vi "Get Frame Signals.vi"(6 "CAN:Frame Type":T1=enum."All", 8 "error in":errorcluster, 9 "Parent Tag":string, 10 "Tree Reference":refnum<vi>, 11 "Frms":refnum<k21>[](array[refnum])) -> (0 "error out":errorcluster, 2 "Tree Reference Out":refnum<vi>)   [LabVIEW 2023, in "J1939 Addon System Explorer.lvlib"]
uses:
  J1939 Addon System Explorer.lvlib
  Types/CAN Frame Filter.ctl
  <resource>/objmgr/xnet.rc
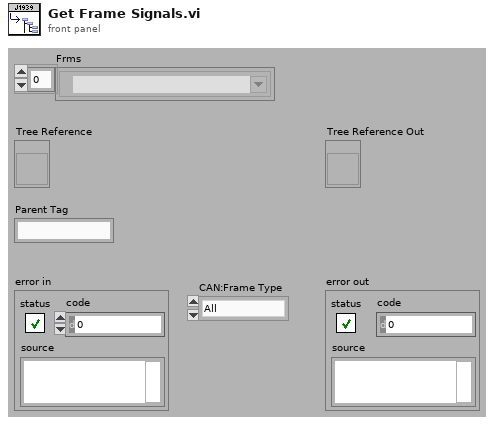
[diagram p1: front panel]
types:
  T1 = typedef "J1939 Addon System Explorer.lvlib/CAN Frame Filter.ctl" = enum16{"Cyclic Data", "Event Data", "Cyclic/Event", "All"}
  T2 = enum16{"open", "replace", "create", "open or create", "replace or create", "replace or create with confirmation"}
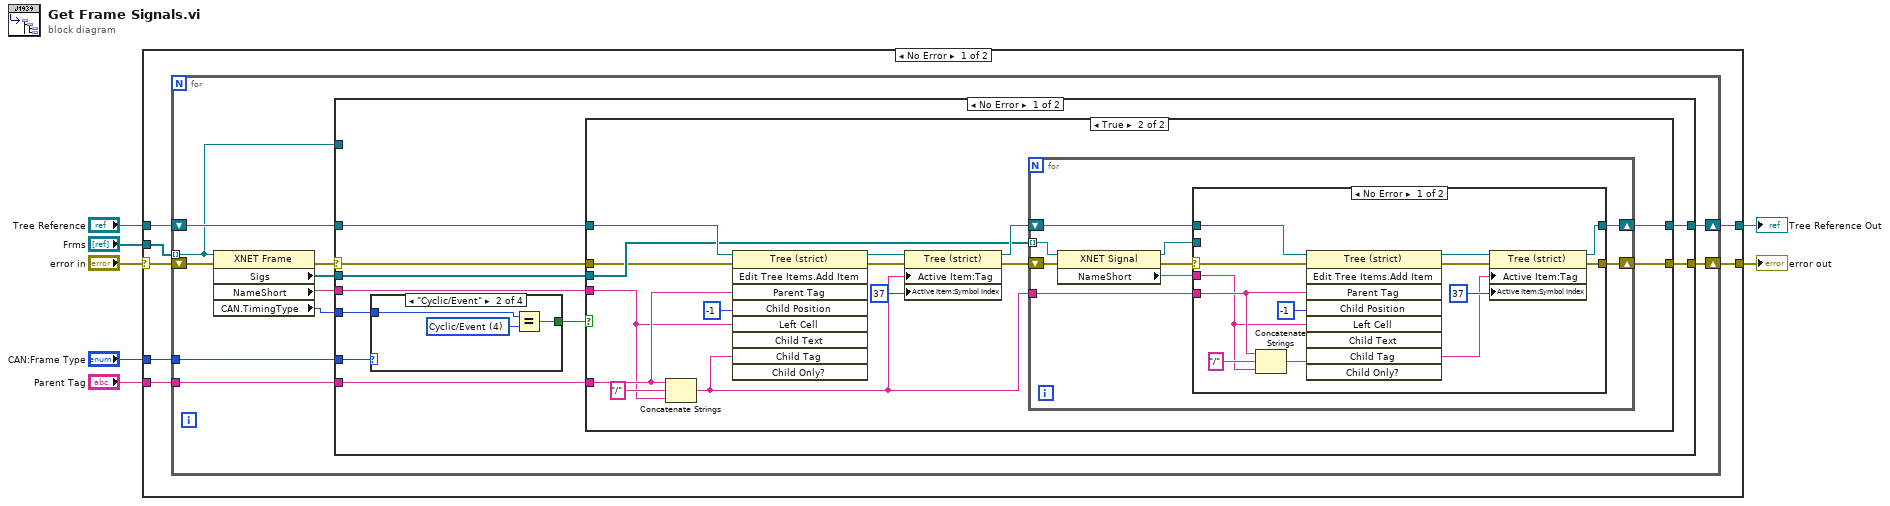
[diagram p0: block diagram]
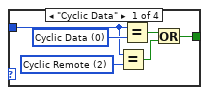
[diagram p2: hidden frame]
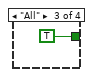
[diagram p3: hidden frame]
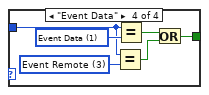
[diagram p4: hidden frame]
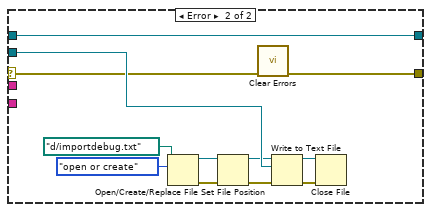
[diagram p6: hidden frame]
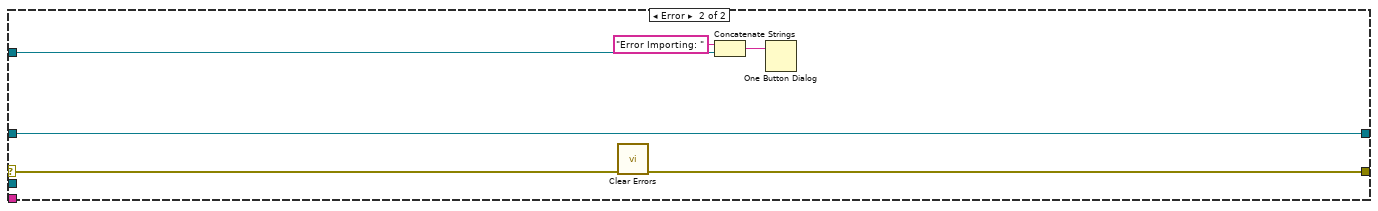
[diagram p7: hidden frame]
diagram:
  n1 = case shown="No Error" "error in" {
    selector: "error in" -> [w11 w109]
    tunnel: [w14 w109] -> w7
    tunnel: "Frms" -> [w9 _]
    tunnel: "Tree Reference" -> [w13 w108]
    tunnel: "Parent Tag" -> [w12 _]
    tunnel: [w10 w108] -> w2
    tunnel: "CAN:Frame Type" -> [w8 _]
    frame No Error {
      n2 = for {
        tunnel: w9 -> [w17] mode=indexing
        shift-right: [w20] -> w14
        shift-left: w11 -> [w25]
        tunnel: w12 -> [w23]
        shift-right: [w22] -> w10
        shift-left: w13 -> [w24]
        tunnel: w8 -> [w16]
        n3 = property class="XNET Frame"(reference=w17, error in=w25) -> (error out=w18:errorcluster, "Sigs"=w21:refnum<k21>[], "NameShort"=w19:string, "CAN.TimingType"=w15:u32)  [unwired: 1 out]
        n4 = case shown="No Error" w18 {
          selector: w18 -> [w29 w104]
          tunnel: w24 -> [w35 w102]
          tunnel: w23 -> [w34 _]
          tunnel: [w33 w102] -> w22
          tunnel: w21 -> [w32 _]
          tunnel: [w31 w103] -> w20
          tunnel: w19 -> [w30 _]
          tunnel: w17 -> [_ w107]
          tunnel: w16 -> [w26 _]
          tunnel: w15 -> [w28 _]
          frame No Error {
            n5 = case shown="\"Cyclic/Event\"" w26 {
              tunnel: w28 -> [w38 w43 _ w49]
              tunnel: [w36 w42 TRUE w47] -> w27
              frame "Cyclic Data" {
                w40 = u32 2 items=["Cyclic Data", "Event Data", "Cyclic Remote", "Event Remote", "Cyclic/Event"] ("CAN:Timing Type")
                w41 = u32 0 items=["Cyclic Data", "Event Data", "Cyclic Remote", "Event Remote", "Cyclic/Event"] ("CAN:Timing Type")
                n6 = Equal?(x=w38, y=w40) -> (x = y?=w39:bool)
                n7 = Equal?(x=w38, y=w41) -> (x = y?=w37:bool)
                n8 = Or(x=w37, y=w39) -> (x .or. y?=w36:bool)
              }
              frame "Cyclic/Event" {
                w44 = u32 4 items=["Cyclic Data", "Event Data", "Cyclic Remote", "Event Remote", "Cyclic/Event"] ("CAN:Timing Type")
                n9 = Equal?(x=w43, y=w44) -> (x = y?=w42:bool)
              }
              frame "All" {
              }
              frame "Event Data" {
                w48 = u32 3 items=["Cyclic Data", "Event Data", "Cyclic Remote", "Event Remote", "Cyclic/Event"] ("CAN:Timing Type")
                w50 = u32 1 items=["Cyclic Data", "Event Data", "Cyclic Remote", "Event Remote", "Cyclic/Event"] ("CAN:Timing Type")
                n10 = Equal?(x=w49, y=w48) -> (x = y?=w46:bool)
                n11 = Equal?(x=w49, y=w50) -> (x = y?=w51:bool)
                n12 = Or(x=w51, y=w46) -> (x .or. y?=w47:bool)
              }
            }
            n13 = case shown="True" w27 {
              tunnel: w35 -> [w53 w68]
              tunnel: w34 -> [_ w65]
              tunnel: [w53 w64] -> w33
              tunnel: w32 -> [_ w57]
              tunnel: [w52 w56] -> w31
              tunnel: w30 -> [_ w55]
              tunnel: w29 -> [w52 w54]
              frame False {
              }
              frame True {
                n14 = Concatenate Strings(w65, "/" ("string"), w55) -> (w58:string)
                n15 = invoke on="Invoke Node" class="Tree (strict)" method="Edit Tree Items.Add Item"(reference=w68, error in=w54, "Parent Tag"=w65, "Child Position"=-1, "Left Cell"=w55, "Child Tag"=w58) -> (reference out=w61:refnum<vi>, error out=w62:errorcluster)  [unwired: 3 in, 7 out]
                n16 = property class="Tree (strict)"(reference=w61, error in=w62, "Active Item:Tag"=w58, "Active Item:Symbol Index"=37) -> (reference out=w59:refnum<vi>, error out=w60:errorcluster)
                n17 = for {
                  tunnel: w57 -> [w70] mode=indexing
                  shift-right: [w72] -> w56
                  shift-left: w60 -> [w77]
                  tunnel: w58 -> [w75]
                  shift-right: [w73] -> w64
                  shift-left: w59 -> [w76]
                  n18 = property class="XNET Signal"(reference=w70, error in=w77) -> (reference out=w69:refnum<k21>, error out=w71:errorcluster, "NameShort"=w74:string)
                  n19 = case shown="No Error" w71 {
                    selector: w71 -> [w78 w99]
                    tunnel: w76 -> [w89 w101]
                    tunnel: w75 -> [w87 _]
                    tunnel: w74 -> [w86 _]
                    tunnel: [w81 w101] -> w73
                    tunnel: [w79 w98] -> w72
                    tunnel: w69 -> [_ w100]
                    frame No Error {
                      n20 = Concatenate Strings(w87, "/" ("string"), w86) -> (w80:string)
                      n21 = invoke on="Invoke Node" class="Tree (strict)" method="Edit Tree Items.Add Item"(reference=w89, error in=w78, "Parent Tag"=w87, "Child Position"=-1, "Left Cell"=w86, "Child Tag"=w80) -> (reference out=w82:refnum<vi>, error out=w83:errorcluster)  [unwired: 3 in, 7 out]
                      n22 = property class="Tree (strict)"(reference=w82, error in=w83, "Active Item:Tag"=w80, "Active Item:Symbol Index"=37) -> (reference out=w81:refnum<vi>, error out=w79:errorcluster)
                    }
                    frame Error {
                      n23 = Open/Create/Replace File(file path (use dialog)=path "d:/importdebug.txt", operation (0:open)=T2."open or create") -> (refnum out=w95:refnum<file>, error out=w96:errorcluster)  [unwired: 4 in, 1 out]
                      n24 = Set File Position(refnum=w95, error in=w96) -> (refnum out=w94:refnum<file>, error out=w93:errorcluster)  [unwired: 2 in]
                      n25 = call <vilib>:"Clear Errors.vi"("error in (no error)"=w99) -> ("error out"=w98:errorcluster)  [unwired: 5 in, 1 out]
                      n26 = Write to Text File(file (use dialog)=w94, text=w100, error in=w93) -> (refnum out=w91:refnum<file>, error out=w92:errorcluster)  [unwired: 1 in, 1 out]
                      n27 = Close File(refnum=w91, error in=w92) -> ()  [unwired: 2 out]
                    }
                  }
                }
              }
            }
          }
          frame Error {
            n28 = call <vilib>:"Clear Errors.vi"("error in (no error)"=w104) -> ("error out"=w103:errorcluster)  [unwired: 5 in, 1 out]
            n29 = Concatenate Strings("Error Importing: " ("string"), w107) -> (w105:string)
            n30 = One Button Dialog(message=w105) -> ()  [unwired: 1 in, 1 out]
          }
        }
      }
    }
    frame Error {
    }
  }
  "error out" <- w7
  "Tree Reference Out" <- w2
